vi "ZCAN_SetResistanceEnable.vi"(8 "error in (no error)":errorcluster caption="错误输入（无错误）", 9 "enable":u32, 10 "can_index":u32, 11 "can_index_handle":u32) -> (0 "error out":errorcluster caption="错误输出", 2 "can_index_handle(out)":u32)   [LabVIEW 2018]
doc: "启用、关闭终端电阻\n在Init 初始化之后， Start 之前使用\n\n适用型号：CANDTU-x00UR、USBCANFD-100U、USBCANFD-200U、USBCANFD-MINI。"
uses:
  zlgcan_demo_CANFDNET_UDP/bin/zlgcan_wrap.dll
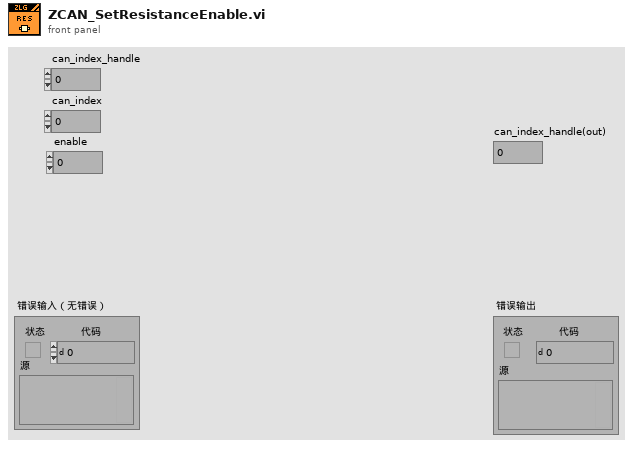
[diagram p1: front panel]
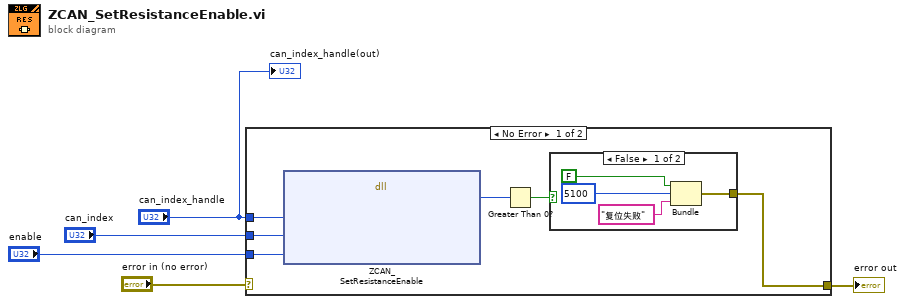
[diagram p0: block diagram]
diagram:
  n1 = case shown="No Error" "error in (no error)" {
    selector: "error in (no error)" -> [_ w16]
    tunnel: [w6 w16] -> w4
    tunnel: "can_index_handle" -> [w11 _]
    tunnel: "can_index" -> [w10 _]
    tunnel: "enable" -> [w9 _]
    frame No Error {
      n2 = dll-call lib="C:/Users/admin/Desktop/zlgcan_demo_CANFDNET_UDP/bin/zlgcan_wrap.dll" fn="ZCAN_SetResistanceEnable"("can_index_handle"=w11, "can_index"=w10, "enable"=w9) -> ("return"=w8:u32)  [unwired: 6 in, 2 out]
      n3 = Greater Than 0?(x=w8) -> (x > 0?=w7:bool)
      n4 = case shown="False" w7 {
        tunnel: [w12 _] -> w6
        frame False {
          n5 = Bundle("status"=FALSE, "code"=5100, "消息"="复位失败") -> (w12:cluster{"status":bool, "code":i32, "消息":string})  [unwired: 1 in]
        }
        frame True {
        }
      }
    }
    frame Error {
    }
  }
  "error out" <- w4
  "can_index_handle(out)" <- "can_index_handle"
